vi "Read Pulse Configuration.vi"(8 "error in (no error)":errorcluster, 11 "Red Pitaya Modulated Digitizer in":refnum<class "Red Pitaya Modulated Digitizer.lvclass">) -> (0 "error out":errorcluster, 2 "Configuration":T1={"Pre-trigger duration"=0.01, "Post-trigger duration"=0.1, "Rate"=1000000.0, "Ranges"=[10.0], "Re-name channels"=[], "Active channels"="0:1", "External clock"=FALSE} {"Rate" format="%#_8pHz"; "Post-trigger duration" format="%#_6ps"; "Pre-trigger duration" format="%#_6ps"; "Ranges" format="%#_6pV"}, 3 "Red Pitaya Modulated Digitizer out":refnum<class "Red Pitaya Modulated Digitizer.lvclass">)   [LabVIEW 2020, in "Red Pitaya Modulated Digitizer.lvclass"]
uses:
  Red Pitaya Modulated Digitizer.lvclass
  Instruments/Pulse Driver/Pusle Driver Configuration.ctl
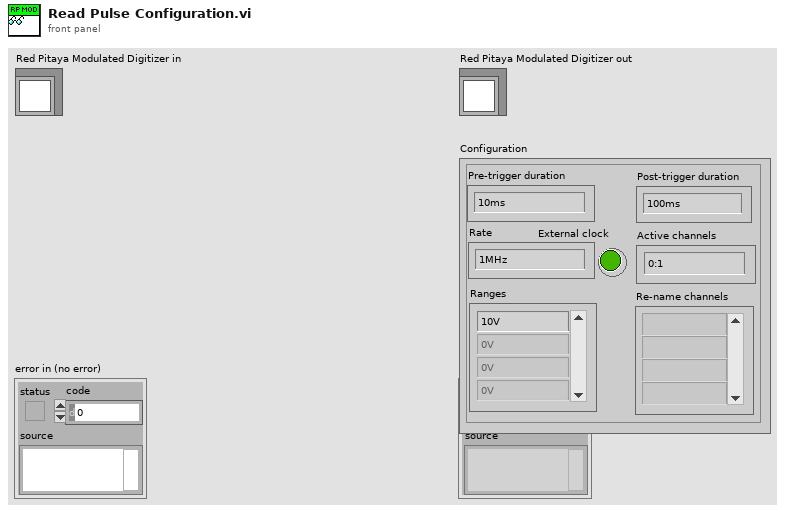
[diagram p1: front panel]
types:
  T1 = typedef "Pusle Driver Configuration.ctl" = cluster{"Pre-trigger duration":dbl, "Post-trigger duration":dbl, "Rate":dbl, "Ranges":dbl[], "Re-name channels":string[], "Active channels":string, "External clock":bool}
  T2 = typedef "RP Modulated Configuration.ctl" = cluster{"Pre-trigger duration":dbl, "Post-trigger duration":dbl, "Rate":dbl, "Ranges":dbl[], "Re-name channels":string[], "Active channels":string, "External clock":bool, "Modulation":T3}
  T3 = typedef "Modulation.ctl" = cluster{"Output delay":dbl, "After delay":bool}
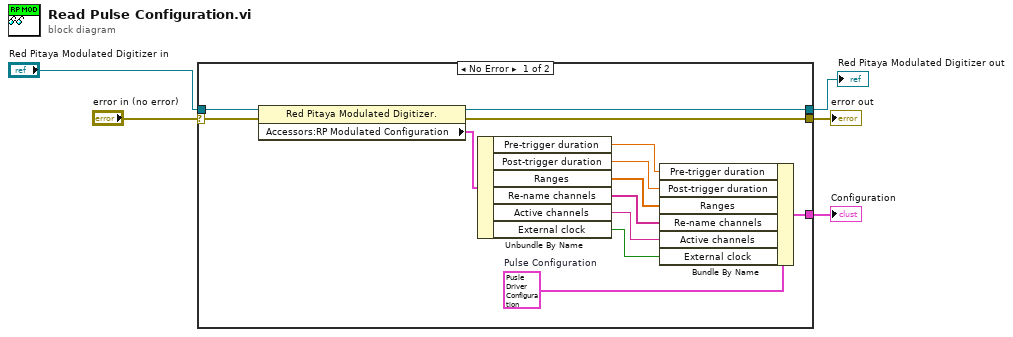
[diagram p0: block diagram]
diagram:
  n1 = case shown="No Error" "error in (no error)" {
    selector: "error in (no error)" -> [w8 w19]
    tunnel: [w9 w19] -> w4
    tunnel: [w7 w20] -> w2
    tunnel: "Red Pitaya Modulated Digitizer in" -> [w6 w20]
    tunnel: [w10 _] -> w1
    frame No Error {
      w11 = T1 {"Pre-trigger duration"=0.01, "Post-trigger duration"=0.1, "Rate"=125000000.0, "Ranges"=[1.0], "Re-name channels"=["V", "I", "Vavg", "Case"], "Active channels"="0:3", "External clock"=FALSE}  # Pulse Configuration
      n2 = property class="Red Pitaya Modulated Digitizer."(reference=w6, error in=w8) -> (reference out=w7:refnum<class "Red Pitaya Modulated Digitizer.lvclass">, error out=w9:errorcluster, "Accessors:RP Modulated Configuration"=w12:T2)
      n3 = Unbundle By Name(w12) -> ("Pre-trigger duration"=w13:dbl, "Post-trigger duration"=w14:dbl, "Ranges"=w15:dbl[], "Re-name channels"=w16:string[], "Active channels"=w17:string, "External clock"=w18:bool)
      n4 = Bundle By Name(cluster=w11, "Pre-trigger duration"=w13, "Post-trigger duration"=w14, "Ranges"=w15, "Re-name channels"=w16, "Active channels"=w17, "External clock"=w18) -> (w10:T1)
    }
    frame Error {
    }
  }
  "error out" <- w4
  "Red Pitaya Modulated Digitizer out" <- w2
  "Configuration" <- w1
